vi "Ballard - 1553 - Clear Database.vi"(8 "error in (no error)":errorcluster, 11 "Node Ptr":u64 format="%.0x") -> (0 "error out":errorcluster)   [LabVIEW 2017, in "Ballard 1553 System Explorer.lvlib"]
uses:
  Ballard 1553 System Explorer.lvlib
  Shared/Controls and Global/Global.vi
  <vilib>/NI Veristand/Custom Device Tools/Custom Device Utility Library/NI VeriStand - Search for All Items by GUID.vi
  <vilib>/NI Veristand/Custom Device Tools/Custom Device Utility Library/NI VeriStand - Search for Item by GUID.vi
  <vilib>/NI VeriStand/Custom Device API/Custom Device API.lvlib
  <vilib>/NI VeriStand/Custom Device Tools/Custom Device Utility Library/Custom Device Utility Library.lvlib
  Shared/Ballard 1553 Shared.lvlib
panel:
  in  "Tag":string
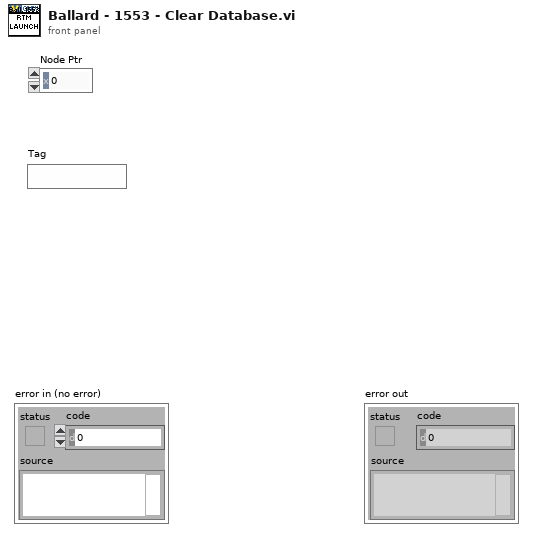
[diagram p1: front panel]
types:
  T1 = typedef "Custom Device API.lvlib/Custom Device Item Ref.ctl" = u64
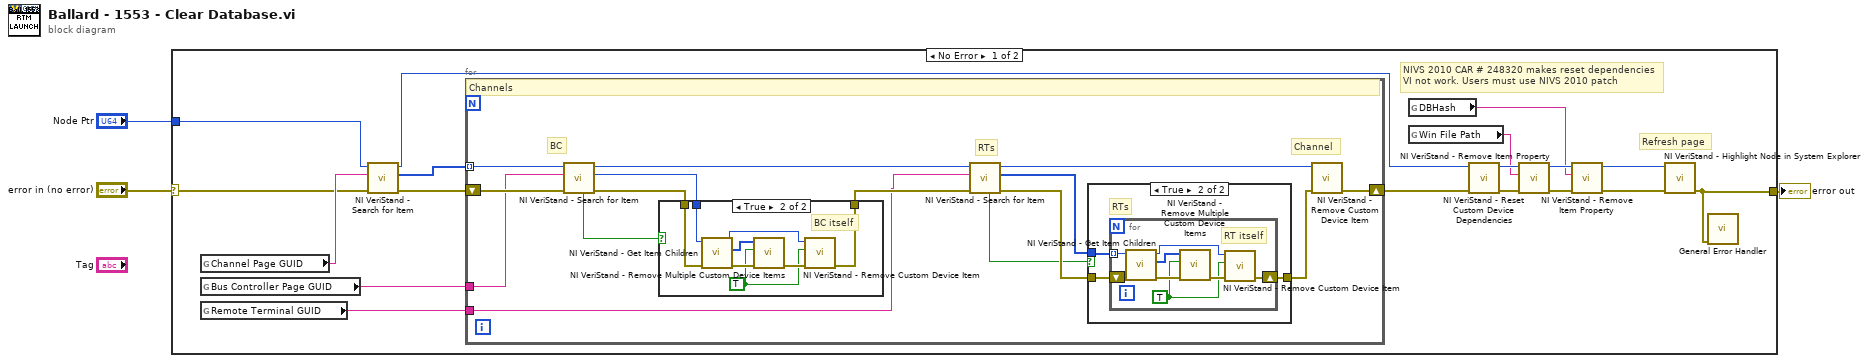
[diagram p0: block diagram]
diagram:
  n1 = case shown="No Error" "error in (no error)" {
    selector: "error in (no error)" -> [w9 w58]
    tunnel: [w18 w58] -> w3
    tunnel: "Node Ptr" -> [w10 _]
    frame No Error {
      # "NIVS 2010 CAR # 248320 makes reset dependencies VI not work. Users must use NIVS 2010 patch"
      # "Refresh page"
      n2 = global read "Global.vi" "Channel Page GUID"() -> (w11:string)
      n3 = global read "Global.vi" "Bus Controller Page GUID"() -> (w6:string)
      n4 = global read "Global.vi" "Remote Terminal GUID"() -> (w4:string)
      n5 = call-poly <vilib>:"NI VeriStand - Search for Item.vi"("error in"=w9, "Item GUID"=w11, "Section Ref in"=w10) -> ("error out"=w8:errorcluster, "Item Refs"=w7:T1[], "Section Ref out"=w5:T1)  [unwired: 5 in, 1 out]
      n6 = for {
        shift-right: [w23] -> w19
        shift-left: w8 -> [w31]
        tunnel: w7 -> [w29] mode=indexing
        tunnel: w6 -> [w30]
        tunnel: w4 -> [w27]
        # "Channel"
        # "RTs"
        # "BC"
        # "Channels"
        n7 = call-poly <vilib>:"NI VeriStand - Search for Item.vi"("error in"=w31, "Item GUID"=w30, "Section Ref in"=w29) -> ("error out"=w35:errorcluster, "Item Ref"=w36:T1, "Section Ref out"=w32:T1, "Found"=w28:bool)  [unwired: 5 in]
        n8 = case shown="True" w28 {
          tunnel: w36 -> [_ w55]
          tunnel: w35 -> [w49 w54]
          tunnel: [w49 w52] -> w34
          frame False {
          }
          frame True {
            w50 = TRUE ("Force Delete (F)")
            # "BC itself"
            n9 = call <vilib>:"NI VeriStand - Get Item Children.vi"("error in (no error)"=w54, "Item Ref in"=w55) -> ("error out"=w57:errorcluster, "Child Refs"=w56:T1[], "Item Ref out"=w51:T1)  [unwired: 6 in, 1 out]
            n10 = call <vilib>:"NI VeriStand - Remove Multiple Custom Device Items.vi"("error in (no error)"=w57, "Force Delete (F)"=w50, "Item Refs in"=w56) -> ("error out"=w53:errorcluster)  [unwired: 7 in, 1 out]
            n11 = call <vilib>:"NI VeriStand - Remove Custom Device Item.vi"("error in (no error)"=w53, "Force Delete (F)"=w50, "Item Ref in"=w51) -> ("error out"=w52:errorcluster)  [unwired: 7 in, 1 out]
          }
        }
        n12 = call-poly <vilib>:"NI VeriStand - Search for Item.vi"("error in"=w34, "Item GUID"=w27, "Section Ref in"=w32) -> ("error out"=w33:errorcluster, "Item Refs"=w25:T1[], "Section Ref out"=w22:T1, "Found"=w26:bool)  [unwired: 5 in]
        n13 = case shown="True" w26 {
          tunnel: w33 -> [w37 w40]
          tunnel: [w37 w39] -> w24
          tunnel: w25 -> [_ w38]
          frame False {
          }
          frame True {
            # "RTs"
            n14 = for {
              shift-right: [w42] -> w39
              shift-left: w40 -> [w47]
              tunnel: w38 -> [w45] mode=indexing
              w43 = TRUE ("Force Delete (F)")
              # "RT itself"
              n15 = call <vilib>:"NI VeriStand - Get Item Children.vi"("error in (no error)"=w47, "Item Ref in"=w45) -> ("error out"=w48:errorcluster, "Child Refs"=w46:T1[], "Item Ref out"=w41:T1)  [unwired: 6 in, 1 out]
              n16 = call <vilib>:"NI VeriStand - Remove Multiple Custom Device Items.vi"("error in (no error)"=w48, "Force Delete (F)"=w43, "Item Refs in"=w46) -> ("error out"=w44:errorcluster)  [unwired: 7 in, 1 out]
              n17 = call <vilib>:"NI VeriStand - Remove Custom Device Item.vi"("error in (no error)"=w44, "Force Delete (F)"=w43, "Item Ref in"=w41) -> ("error out"=w42:errorcluster)  [unwired: 7 in, 1 out]
            }
          }
        }
        n18 = call <vilib>:"NI VeriStand - Remove Custom Device Item.vi"("error in (no error)"=w24, "Item Ref in"=w22) -> ("error out"=w23:errorcluster)  [unwired: 8 in, 1 out]
      }
      n19 = global read "Global.vi" "DBHash"() -> (w13:string)
      n20 = global read "Global.vi" "Win File Path"() -> (w12:string)
      n21 = call <vilib>:"NI VeriStand - Reset Custom Device Dependencies.vi"("error in (no error)"=w19, "Device Ref in"=w5) -> ("error out"=w21:errorcluster, "Device Ref out"=w20:T1)  [unwired: 8 in]
      n22 = call <vilib>:"NI VeriStand - Remove Item Property.vi"("error in (no error)"=w21, "Property Name"=w12, "Item Ref in"=w20) -> ("error out"=w17:errorcluster, "Item Ref out"=w16:T1)  [unwired: 6 in, 1 out]
      n23 = call <vilib>:"NI VeriStand - Remove Item Property.vi"("error in (no error)"=w17, "Property Name"=w13, "Item Ref in"=w16) -> ("error out"=w15:errorcluster, "Item Ref out"=w14:T1)  [unwired: 6 in, 1 out]
      n24 = call <vilib>:"NI VeriStand - Highlight Node in System Explorer.vi"("error in (no error)"=w15, "Item Ref in"=w14) -> ("error out"=w18:errorcluster)  [unwired: 8 in, 1 out]
      n25 = call <vilib>:"General Error Handler.vi"("error in (no error)"=w18) -> ()  [unwired: 10 in, 5 out]
    }
    frame Error {
    }
  }
  "error out" <- w3
